vi "Pattern_to_YAML.vi"(2 "Ym String (csv)":string="13.84,  23.78,  13.79,  13.83,  13.75,  13.79,  13.74,  13.68", 3 "Xm String (csv)":string="21.72,  44.87,  68.20,  91.45, 114.72, 137.87, 160.97, 184.04", 4 "Pattern Definition":T1={"Spot pitch (pixels)"=31.3, "Tilt Angle (deg)"=0.0, "Horizontal Offset (pixels)"=-3.0, "Vertical Offset (pixels)"=-32.0, "# Horizontal Spots"=6, "# Vertical Spots"=4, "Spot size (pixels)"=31.3, "Darken center spot"=TRUE, "Exact Phase Formula"=TRUE, "phase wrapping"=TRUE, "Set Focus (mm)"=32.0, "Add phase"=4.0, "phase_factor"=56.0, "Steering LW"=1.0, "Steering vmax"=60.0, "phase_overshoot"=TRUE, "Focal shift param"=0.0, "x0 focal shift"=0.0, "y0 focal shift"=0.0, "hv_steering"=TRUE, "fixed"=FALSE, "Pad"=0.0, "dark_all"=FALSE, "nospot"=FALSE, "Laser wavelength"=6.28e-07} {"Laser wavelength" min=0.0 max=500.0 format="%^#.3e"; "Pad" min=0.0 max=500.0 step=1.0 format="%#.0g"; "y0 focal shift" min=0.0 max=500.0 format="%#.3g"; "x0 focal shift" min=0.0 max=500.0 format="%#.3g"; "Focal shift param" min=0.0 max=500.0 format="%#.3g"; "Steering vmax" min=0.0 max=500.0 format="%#.3g"; "Steering LW" min=0.0 max=500.0 format="%#.3g"; "phase_factor" min=0.0 max=500.0 format="%#.3f"; "Add phase" min=0.0 max=500.0 format="%#.3f"; "Set Focus (mm)" min=0.0 max=500.0 format="%#.3g"; "Spot size (pixels)" min=1.0 format="%.2g"; "# Vertical Spots" min=1 step=1; "# Horizontal Spots" min=1 step=1; "Vertical Offset (pixels)" format="%.2f"; "Horizontal Offset (pixels)" format="%.2f"; "Tilt Angle (deg)" min=-90.0 max=90.0 format="%.2g"; "Spot pitch (pixels)" min=1.0 format="%.2g"}) -> (0 "Result":string)   [LabVIEW 2011]
uses:
  Periodic Spot Pattern Parameters.ctl
  Periodic Spot Pattern Parameters2.ctl
panel:
  in  "Debug":bool
  in  "center_spot (to be darkened)":u16=4
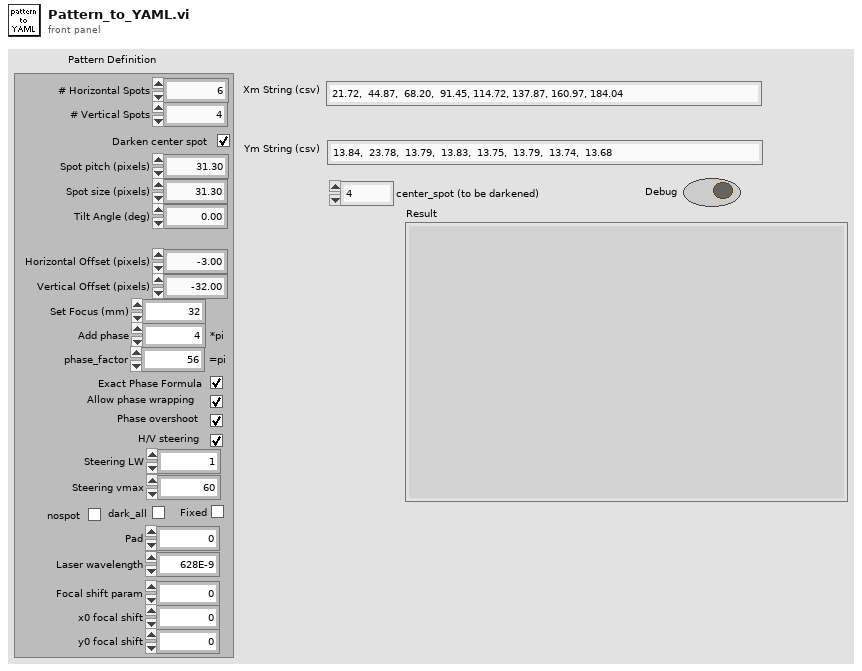
[diagram p1: front panel]
types:
  T1 = typedef "Periodic Spot Pattern Parameters.ctl" = cluster{"Spot pitch (pixels)":dbl, "Tilt Angle (deg)":dbl, "Horizontal Offset (pixels)":dbl, "Vertical Offset (pixels)":dbl, "# Horizontal Spots":u32, "# Vertical Spots":u32, "Spot size (pixels)":dbl, "Darken center spot":bool, "Exact Phase Formula":bool, "phase wrapping":bool, "Set Focus (mm)":T2, "Add phase":dbl, "phase_factor":dbl, "Steering LW":T2, "Steering vmax":T2, "phase_overshoot":bool, "Focal shift param":T2, "x0 focal shift":T2, "y0 focal shift":T2, "hv_steering":bool, "fixed":bool, "Pad":T2, "dark_all":bool, "nospot":bool, "Laser wavelength":dbl}
  T2 = typedef "Periodic Spot Pattern Parameters2.ctl" = dbl
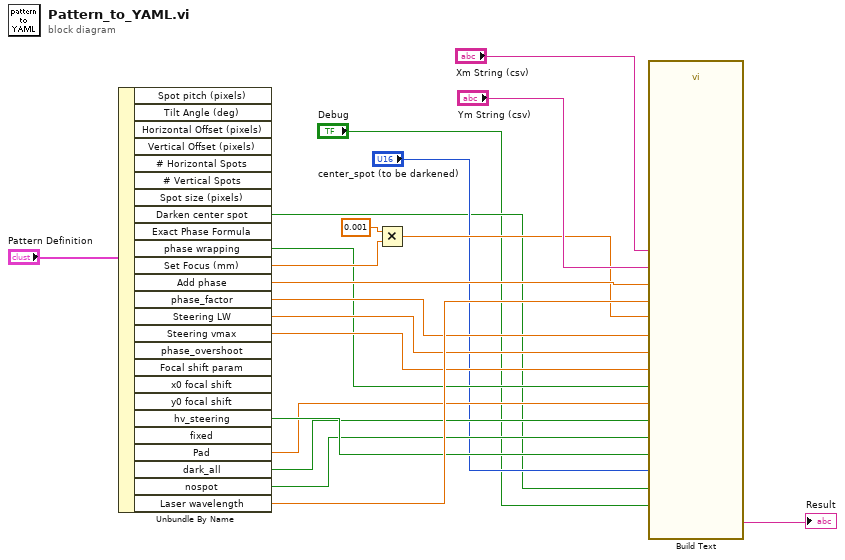
[diagram p0: block diagram]
diagram:
  n1 = Unbundle By Name("Pattern Definition") -> ("Darken center spot"=w3:bool, "phase wrapping"=w7:bool, "Set Focus (mm)"=w14:T2, "Add phase"=w17:dbl, "phase_factor"=w12:dbl, "Steering LW"=w11:T2, "Steering vmax"=w10:T2, "hv_steering"=w9:bool, "Pad"=w8:T2, "dark_all"=w5:bool, "nospot"=w6:bool, "Laser wavelength"=w16:dbl)  [unwired: 13 out]
  n2 = Multiply(x=T2 0.001, y=w14) -> (x*y=w13:T2)
  n3 = call "Build Text"("Xm"="Xm String (csv)", "Ym"="Ym String (csv)", "phi_max"=w17, "wl"=w16, "f"=w13, "phase_factor"=w12, "center_spot"="center_spot (to be darkened)", "darken_cspot"=w3, "lw"=w11, "vmax"=w10, "PhWrap"=w7, "pad"=w8, "dark_all"=w5, "nospot"=w6, "steer_horiz"=w9, "debug"="Debug") -> ("Result"=→"Result":string)  [unwired: 10 in, 1 out]
